vi "Trav_3D_volume.vi"(3 "Simulate/Run":T1, 5 "Traverse line":T2 {"Row Duration (mins)" format="%#.1f"; "Row No" min=0; "Trace Gas Concentration (%)" min=0.0 format="%#.2f"; "Emission Rate (l/min)" format="%#.2f"; "Tunnel Speed" format="%#.2f"; "Start X" format="%#.2f"; "Start Y" format="%#.2f"; "Start Z" format="%#.2f"; "End X" format="%#.2f"; "End Y" format="%#.2f"; "End Z" format="%#.2f"; "Averaging time (min)" min=0.0 format="%#.2f"}) -> (0 "Error Messages":string, 1 "Status":T5, 2 "Traverse line Out":T2 {"Row Duration (mins)" format="%#.1f"; "Row No" min=0; "Trace Gas Concentration (%)" min=0.0 format="%#.2f"; "Emission Rate (l/min)" format="%#.2f"; "Tunnel Speed" format="%#.2f"; "Start X" format="%#.2f"; "Start Y" format="%#.2f"; "Start Z" format="%#.2f"; "End X" format="%#.2f"; "End Y" format="%#.2f"; "End Z" format="%#.2f"; "Averaging time (min)" min=0.0 format="%#.2f"})   [LabVIEW 2011]
uses:
  Gen Trav/Multi_Run_Status.ctl
  Gen Trav/Traverse_cluster.ctl
  Gen Trav/Spacing.ctl
  Controls/Multi_run_mode.ctl
  Controls/User_Specific_mode.ctl
  Controls/Save_Data.ctl
  Controls/Setup.ctl
  ADAM Client/Sub VIs/ADAM Controls/Traverse_Level_State.ctl
  Controls/Overhead.ctl
  Globals/Trav_pos_global.vi
  Globals/Meas_global.vi
panel:
  out "Pause message":string
  in  "Pause":bool
  out "Current position":dbl[](array[numeric]) format="%.2f"
  in  "stop":bool
  in  "Array of Positions":dbl[][](array[numeric]) format="%.2f"
  out "Abcissa copy":string="Y (mm)"
  out "Abcissa":string="Y (mm)"
  in  "Plot 1":i32[](listbox)=[1]
  out "Started Profile at:":string="16/9/98 12:33"
  out "Currently on point":i32=9
  out "U":cluster{dbl[], dbl[]}[](graph)
  out "% u'/U":cluster{dbl[], dbl[]}[](graph)
  # "X           Y            Z"
  # "Start"
  # "End"
  # "X           Y            Z"
  # "Start"
  # "End"
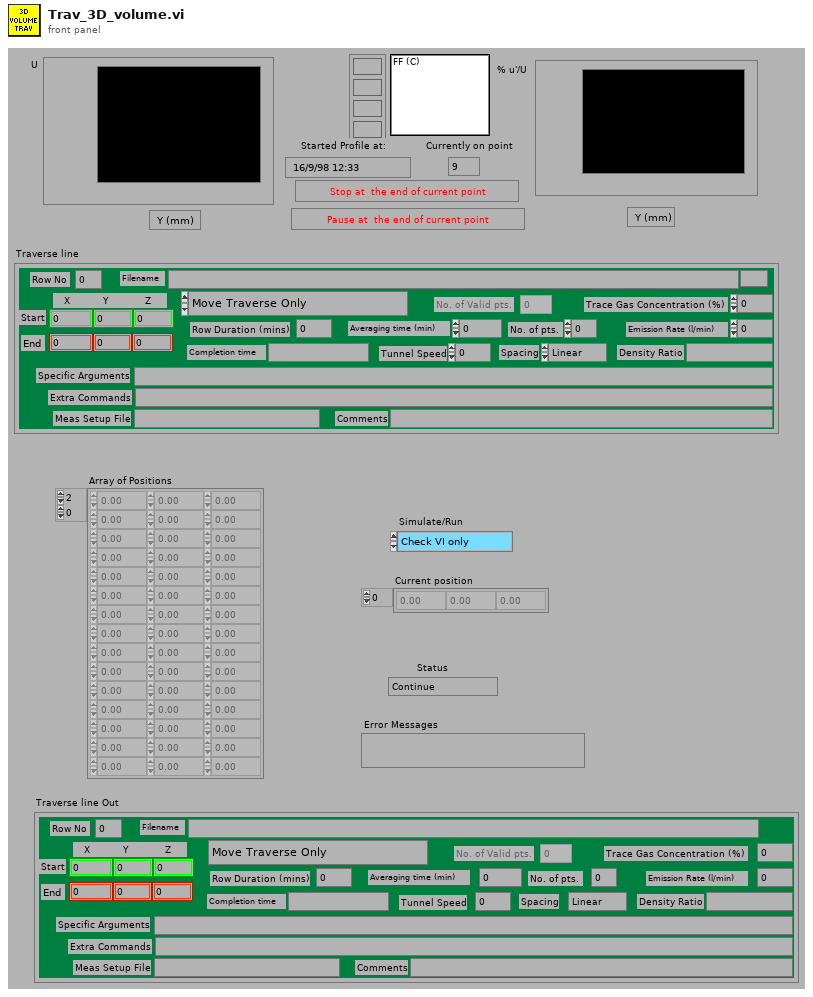
[diagram p1: front panel]
types:
  T1 = typedef "User_Specific_mode.ctl" = enum16{"Check VI only", "Run VI"}
  T2 = typedef "Traverse_cluster.ctl" = cluster{"Start X":dbl, "Start Y":dbl, "Start Z":dbl, "End X":dbl, "End Y":dbl, "End Z":dbl, "No. of pts.":i32, "Spacing":T3, "Filename":path, "Tunnel Speed":dbl, "Averaging time (min)":dbl, "Extra Commands":string, "Specific Arguments":string, "Emission Rate (l/min)":dbl, "Trace Gas Concentration (%)":dbl, "Density Ratio":string, "Comments":string, "Row No":i32, "Row Type Selector":T4, "Completion time":string, "Row Duration (mins)":dbl, "No. of Valid pts.":i32, "Meas Setup File":string}
  T3 = typedef "Spacing.ctl" = enum16{"Linear", "Log", "Gauss", "Specified", "N/A"}
  T4 = typedef "Multi_run_mode.ctl" = enum16{"Move Traverse Only", "Set Tunnel Speed Only", "Set Source Only", "Set Measurement Conditions", "Single Measurement", "Vertical Profile", "Lateral Profile", "Longitudinal Profile", "Explore Volume", "Multi-Axis Profile", "Auto Calibrate", "Meas Fast FID Bkgnd", "Check Beam Power", "Scanning Valve Measurement", "Run VI Named:", "Set ADAM Ch", "Wait (minutes)", "Send Message", "Synchronize With:", "Fall Back to this Row", "Turn Off Row Repeating", "Blank Row", "Traverse 3D Volume"}
  T5 = typedef "Multi_Run_Status.ctl" = enum16{"Continue", "Jump to Next Point", "Jump to Next Row", "Jump To Fall Back", "Terminate Run"}
  T6 = typedef "Save_Data.ctl" = enum16{"Save No Data", "Save Data"}
  T7 = typedef "Setup.ctl" = enum16{"Run Program", "Show Setup", "Save Current Setup", "Setup Front Panel"}
  T8 = typedef "Traverse_Level_State.ctl" = enum16{"Running", "Complete"}
  T9 = typedef "Overhead.ctl" = enum16{"Update total times", "Read Current Overhead", "Re Scale totals to 3 hrs", "Initialise totals to 3hr"}
  T10 = typedef "Status_Cluster.ctl" = cluster{"Status":T5, "Error Type":string, "Error Description":string}
  T11 = typedef "Velocity_cluster.ctl" = cluster{"Name":string, "U":dbl, "u^2":dbl, "u^3/(u^2)^(1.5)":dbl, "u^4/(u^2)^2 -3":dbl, "% u'/U":dbl, "Mean % Err":dbl, "u^4":dbl}
  T12 = typedef "Analysis_type_cluster.ctl" = cluster{"Analysis type":T13, "Indicies":i32[], "Name":string, "Inst Array":T14, "Info index":i32}
  T13 = typedef "Analysis_type_Enum.ctl" = enum16{"Slow Response", "Fast Response", "Weighted Fast Response", "Fast FID", "Weighted Fast FID", "Cross Wire", "Weighted Cross Wire", "Weighted LDA"}
  T14 = typedef "Instrument_Array.ctl" = enum16{"PWA", "LDA", "Analogue"}
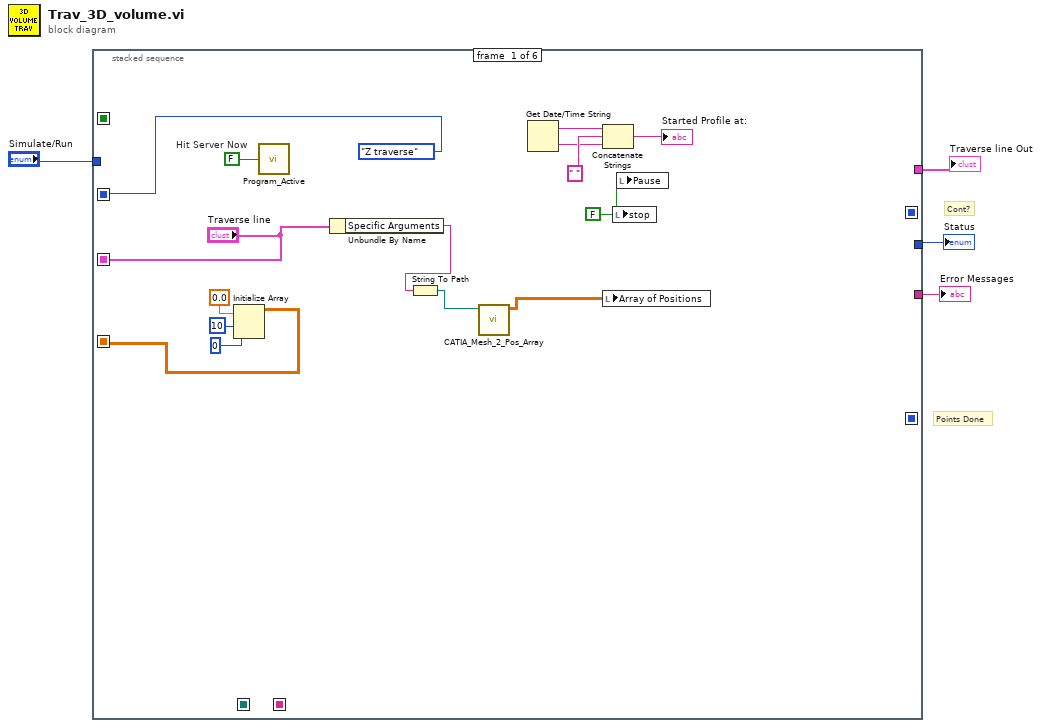
[diagram p0: block diagram]
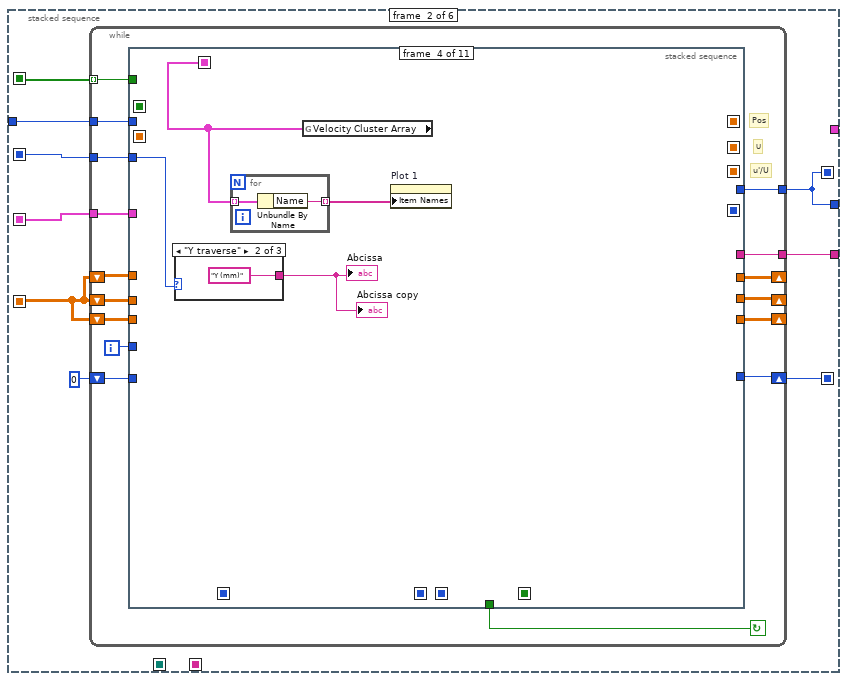
[diagram p2: hidden frame]
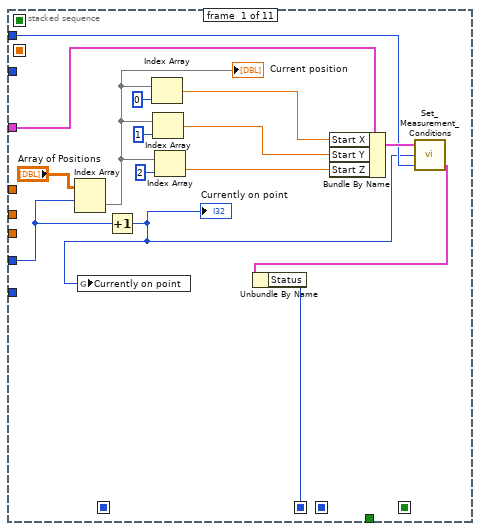
[diagram p3: hidden frame]
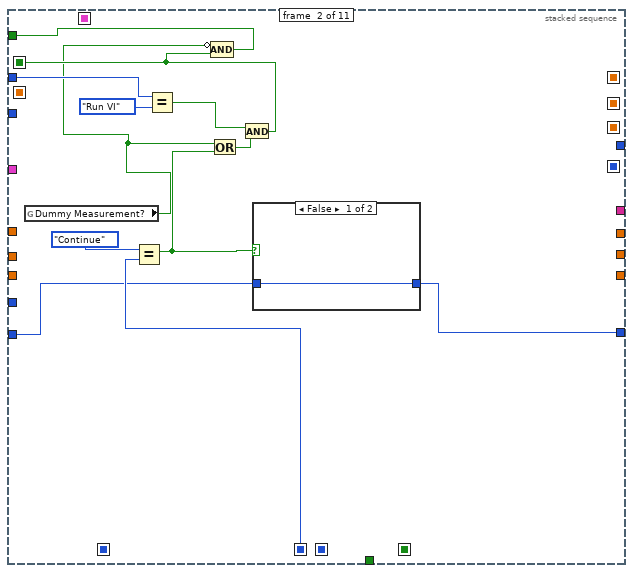
[diagram p4: hidden frame]
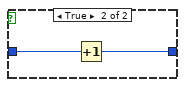
[diagram p5: hidden frame]
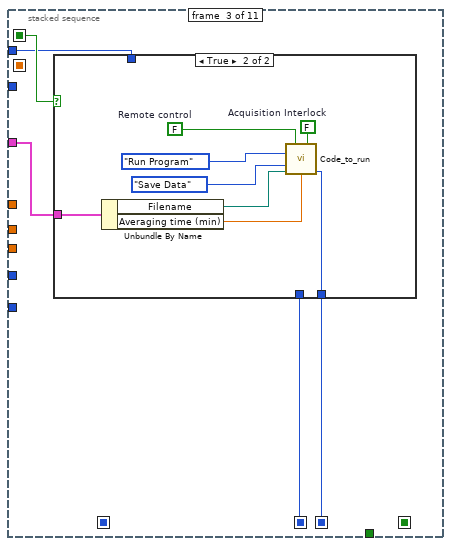
[diagram p6: hidden frame]
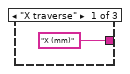
[diagram p8: hidden frame]
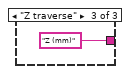
[diagram p9: hidden frame]
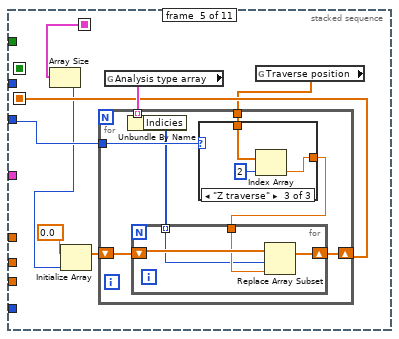
[diagram p10: hidden frame]
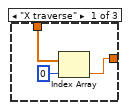
[diagram p11: hidden frame]
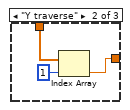
[diagram p12: hidden frame]
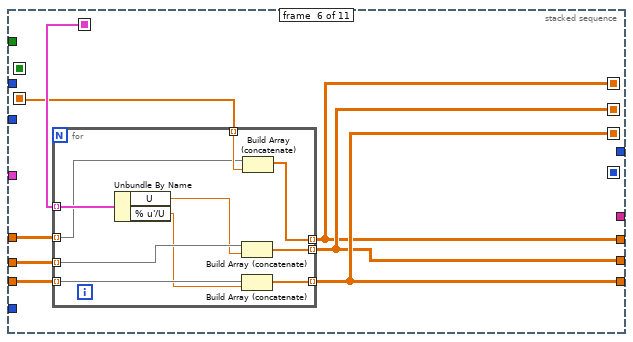
[diagram p13: hidden frame]
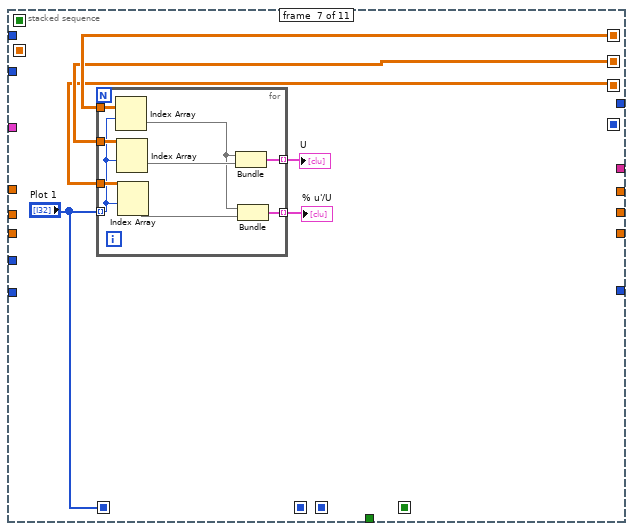
[diagram p14: hidden frame]
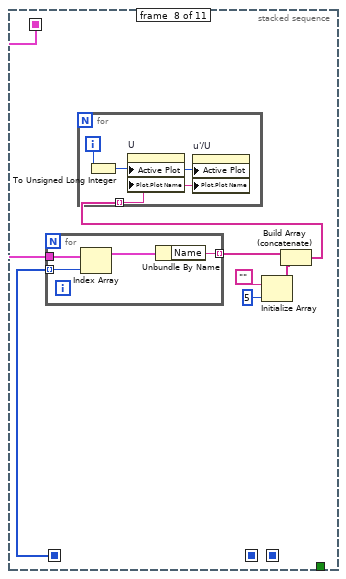
[diagram p15: hidden frame]
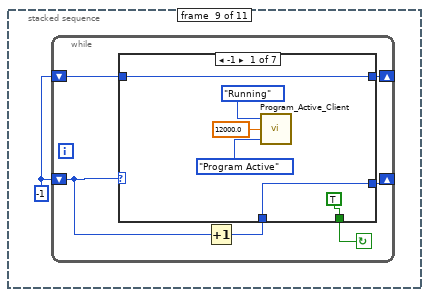
[diagram p16: hidden frame]
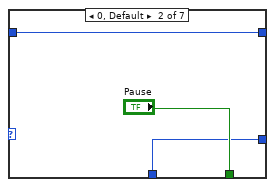
[diagram p17: hidden frame]
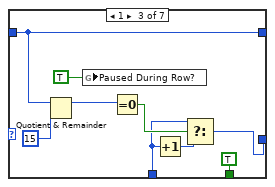
[diagram p18: hidden frame]
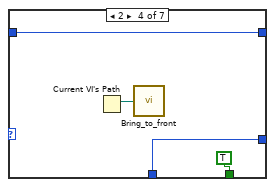
[diagram p19: hidden frame]
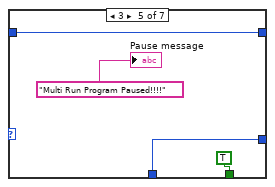
[diagram p20: hidden frame]
diagram:
  # "Points Done"
  # "Cont?"
  n1 = stacked-sequence {
    seq-local: [w12 _ _ _ _ _] -> [_ w27 _ _ _ _]
    seq-local: [enum16{"X traverse", "Y traverse", "Z traverse"}."Z traverse" ("Axis Traversed") _ _ _ _ _] -> [_ w28 _ _ _ _]
    seq-local: [_ _ w277 _ _ _] -> [_ _ _ _ w301 _]
    seq-local: [_ _ _ w284 _ _] -> [_ _ _ _ w300 _]
    seq-local: [_ w26 _ _ _ _] -> [_ _ _ _ _ _]
    seq-local: [_ w24 _ _ _ _] -> [_ _ _ w281 w299 _]
    seq-local: [_ w22 _ _ _ _] -> [_ _ _ _ _ w306]
    seq-local: ["Traverse line" _ _ _ _ _] -> [_ w21 _ _ _ w308]
    tunnel: [_ w26 _ _ _ _] -> w2
    tunnel: [_ _ _ _ _ w318] -> w4
    tunnel: "Simulate/Run" -> [_ w25 _ _ _ w317]
    tunnel: [_ w20 _ _ _ _] -> w1
    frame #0 {
      w10 = FALSE ("stop")
      w11 = FALSE  # Hit Server Now
      n2 = Initialize Array(0.0, 10, 0) -> (w12:dbl[][])
      n3 = call "Program_Active.vi"("Hit Server Now"=w11) -> ()
      n4 = Unbundle By Name("Traverse line") -> ("Specific Arguments"=w6:string)
      n5 = String To Path(string=w6) -> (path=w5:path)
      n6 = call "CATIA_Mesh_2_Pos_Array.vi"("Catia Mesh File"=w5) -> ("Array of Positions"=w8:dbl[][])  [unwired: 10 in]
      n7 = Get Date/Time String() -> (date string=w18:string, time string=w17:string)  [unwired: 3 out]
      n8 = Concatenate Strings(w18, " ", w17) -> (→"Started Profile at:":string)
      n9 = local write "Array of Positions"(w8) -> ()
      n10 = local write "stop"(w10) -> ()
      n11 = local write "Pause"(w10) -> ()
    }
    frame #1 {
      n12 = while {
        shift-left: 0 -> [w31]
        shift-right: [w30] -> w22
        tunnel: [w32] -> w24 mode=indexing
        tunnel: w21 -> [w33]
        tunnel: w25 -> [w34]
        tunnel: [w35] -> w26
        shift-left: w27 -> [w38]
        shift-right: [w37] -> _
        tunnel: w28 -> [w39]
        shift-left: w27 -> [w41]
        shift-right: [w40] -> _
        shift-left: w27 -> [w43]
        shift-right: [w42] -> _
        tunnel: [w29] -> w20
        i -> [w44]
        stop <- w36 continue-if-true
        # "Pos"
        # "U"
        # "u'/U"
        n13 = stacked-sequence {
          seq-local: [_ _ _ _ w103 _ _ _ _ _ _] -> [_ _ _ _ _ w128 _ _ _ _ _]
          seq-local: [_ _ _ w92 _ _ _ _ _ _ _] -> [_ _ _ _ w102 w131 _ w159 _ _ _]
          seq-local: [_ _ _ _ _ w126 _ _ _ _ _] -> [_ _ _ _ _ _ w149 _ _ _ _]
          seq-local: [_ _ _ _ _ w129 _ _ _ _ _] -> [_ _ _ _ _ _ w148 _ _ _ _]
          seq-local: [_ _ _ _ _ w130 _ _ _ _ _] -> [_ _ _ _ _ _ w147 _ _ _ _]
          seq-local: [_ _ _ _ _ _ "Plot 1" _ _ _ _] -> [_ _ _ _ _ _ _ w165 _ _ _]
          seq-local: [_ _ w78 _ _ _ _ _ _ _ _] -> [_ _ _ _ _ _ _ _ _ w223 _]
          seq-local: [w49 _ _ _ _ _ _ _ _ _ _] -> [_ w69 w76 _ _ _ _ _ _ _ _]
          seq-local: [_ w62 _ _ _ _ _ _ _ _ _] -> [_ _ w77 _ _ _ _ _ _ _ _]
          seq-local: [_ _ _ _ _ _ _ _ _ w218 _] -> [_ _ _ _ _ _ _ _ _ _ w239]
          seq-local: [_ _ _ _ _ _ _ _ _ w217 _] -> [_ _ _ _ _ _ _ _ _ _ w233]
          tunnel: w44 -> [w46 _ _ _ _ _ _ _ _ w229 w236]
          tunnel: w43 -> [_ _ _ _ _ w133 _ _ _ _ _]
          tunnel: [_ _ _ _ _ w129 _ _ _ _ _] -> w42
          tunnel: w41 -> [_ _ _ _ _ w132 _ _ _ _ _]
          tunnel: [_ _ _ _ _ w130 _ _ _ _ _] -> w40
          tunnel: w39 -> [_ _ _ w90 w104 _ _ _ _ _ _]
          tunnel: w38 -> [_ _ _ _ _ w127 _ _ _ _ _]
          tunnel: [_ _ _ _ _ w126 _ _ _ _ _] -> w37
          tunnel: [_ _ _ _ _ _ _ _ _ w218 _] -> w36
          tunnel: w33 -> [w53 _ w79 _ _ _ _ _ _ _ w237]
          tunnel: [_ _ _ _ _ _ _ _ _ _ w235] -> w35
          tunnel: w34 -> [w51 w71 w75 _ _ _ _ _ _ _ w238]
          tunnel: [_ w61 _ _ _ _ _ _ _ _ _] -> w32
          tunnel: w31 -> [_ w66 _ _ _ _ _ _ _ _ _]
          tunnel: [_ w65 _ _ _ _ _ _ _ _ _] -> w30
          tunnel: [_ _ _ _ _ _ _ _ _ _ w234] -> w29
          frame #0 {
            n14 = Index Array(array="Array of Positions", index (row)=w46) -> (element=w45:dbl[])  [unwired: 1 in]
            "Current position" <- w45
            n15 = Increment(x=w46) -> (x+1=w48:i32)
            "Currently on point" <- w48
            n16 = global write "Trav_pos_global.vi" "Currently on point"(w48) -> ()
            n17 = Index Array(array=w45, index=0 ("Index")) -> (element=w56:dbl)
            n18 = Index Array(array=w45, index=1 ("Index")) -> (element=w55:dbl)
            n19 = Index Array(array=w45, index=2 ("Index")) -> (element=w54:dbl)
            n20 = Bundle By Name(cluster=w53, "Start X"=w56, "Start Y"=w55, "Start Z"=w54) -> (w52:T2)
            n21 = call "Set_Measurement_Conditions.vi"("Simulate/Run"=w51, "Currently on Point"=w48, "Traverse line"=w52) -> ("Status Cluster"=w50:T10)  [unwired: 2 out]
            n22 = Unbundle By Name(w50) -> ("Status"=w49:T5)
          }
          frame #1 {
            n23 = global read "Trav_pos_global.vi" "Dummy Measurement?"() -> (w60:bool)
            n24 = Equal?(x=Multi_Run_Status."Continue" ("Status"), y=w69) -> (x = y?=w64:bool)
            n25 = Equal?(x=w71, y=User_Specific_mode."Run VI" ("Simulate/Run")) -> (x = y?=w67:bool)
            n26 = Or(x=w60, y=w64) -> (x .or. y?=w63:bool)
            n27 = And(x=w67, y=w63) -> (x .and. y?=w62:bool)
            n28 = Compound Arithmetic op=AND(invert w60, w62) -> (w61:bool)
            n29 = case shown="False" w64 {
              tunnel: w66 -> [w72 w74]
              tunnel: [w72 w73] -> w65
              frame False {
              }
              frame True {
                n30 = Increment(x=w74) -> (x+1=w73:i32)
              }
            }
          }
          frame #2 {
            n31 = case shown="True" w77 {
              tunnel: w79 -> [_ w88]
              tunnel: [w80 w87] -> w78
              tunnel: w76 -> [w80 _]
              tunnel: w75 -> [_ _]
              frame False {
              }
              frame True {
                w83 = FALSE  # Acquisition Interlock
                w86 = FALSE  # Remote control
                n32 = Unbundle By Name(w88) -> ("Filename"=w84:path, "Averaging time (min)"=w85:dbl)
                n33 = call "Code_to_run.vi"("Acquisition Interlock"=w83, "setup"=Setup."Run Program", "Remote control"=w86, "File"=Save_Data."Save Data", "Results Filename"=w84, "Averaging time (min)"=w85) -> ("Status"=w87:T5)  [unwired: 5 in, 4 out]
              }
            }
          }
          frame #3 {
            n34 = case shown="\"Y traverse\"" w90 {
              tunnel: ["X (mm)" "Y (mm)" "Z (mm)"] -> w89
              frame "X traverse" {
              }
              frame "Y traverse" {
              }
              frame "Z traverse" {
              }
            }
            "Abcissa" <- w89
            "Abcissa copy" <- w89
            n35 = global read "Meas_global.vi" "Velocity Cluster Array"() -> (w92:T11[])
            n36 = for {
              tunnel: w92 -> [w97] mode=indexing
              tunnel: [w96] -> w91 mode=indexing
              n37 = Unbundle By Name(w97) -> ("Name"=w96:string)
            }
            n38 = property on="Plot 1" class="LstBox (strict)"("Item Names"=w91) -> ()  [unwired: 2 in, 2 out]
          }
          frame #4 {
            n39 = Array Size(array=w102) -> (size(s)=w101:i32)
            n40 = Initialize Array(0.0, w101) -> (w99:dbl[])
            n41 = global read "Meas_global.vi" "Analysis type array"() -> (w105:T12[])
            n42 = global read "Trav_pos_global.vi" "Traverse position"() -> (w98:dbl[])
            n43 = for {
              shift-right: [w109] -> w103
              shift-left: w99 -> [w110]
              tunnel: w105 -> [w112] mode=indexing
              tunnel: w104 -> [w111]
              tunnel: w98 -> [w106]
              n44 = Unbundle By Name(w112) -> ("Indicies"=w107:i32[])
              n45 = case shown="\"Z traverse\"" w111 {
                tunnel: [w118 w121 w123] -> w108
                tunnel: w106 -> [w119 w120 w124]
                frame "X traverse" {
                  n46 = Index Array(array=w119, index=0) -> (element=w118:dbl)
                }
                frame "Y traverse" {
                  n47 = Index Array(array=w120, index=1) -> (element=w121:dbl)
                }
                frame "Z traverse" {
                  n48 = Index Array(array=w124, index=2) -> (element=w123:dbl)
                }
              }
              n49 = for {
                shift-right: [w115] -> w109
                shift-left: w110 -> [w116]
                tunnel: w108 -> [w114]
                tunnel: w107 -> [w113] mode=indexing
                n50 = Replace Array Subset(array=w116, new element=w114, index=w113) -> (w115:dbl[])
              }
            }
          }
          frame #5 {
            n51 = for {
              tunnel: w133 -> [w143] mode=indexing
              tunnel: [w141] -> w129 mode=indexing
              tunnel: w132 -> [w140] mode=indexing
              tunnel: [w138] -> w130 mode=indexing
              tunnel: w131 -> [w137] mode=indexing
              tunnel: w128 -> [w136] mode=indexing
              tunnel: w127 -> [w135] mode=indexing
              tunnel: [w134] -> w126 mode=indexing
              n52 = Unbundle By Name(w137) -> ("U"=w142:dbl, "% u'/U"=w139:dbl)
              n53 = Build Array (concatenate)(w143, w142) -> (w141:dbl[])
              n54 = Build Array (concatenate)(w140, w139) -> (w138:dbl[])
              n55 = Build Array (concatenate)(w135, w136) -> (w134:dbl[])
            }
          }
          frame #6 {
            n56 = for {
              tunnel: "Plot 1" -> [w150] mode=indexing
              tunnel: w149 -> [w158]
              tunnel: w148 -> [w157]
              tunnel: w147 -> [w156]
              tunnel: [w152] -> w146 mode=indexing
              tunnel: [w151] -> w145 mode=indexing
              n57 = Index Array(array=w158, index (row)=w150) -> (element=w154:dbl[])  [unwired: 1 in]
              n58 = Index Array(array=w157, index (row)=w150) -> (element=w155:dbl[])  [unwired: 1 in]
              n59 = Index Array(array=w156, index (row)=w150) -> (element=w153:dbl[])  [unwired: 1 in]
              n60 = Bundle(w154, w155) -> (w151:cluster{dbl[], dbl[]})  [unwired: 1 out]
              n61 = Bundle(w154, w153) -> (w152:cluster{dbl[], dbl[]})  [unwired: 1 out]
            }
            "U" <- w145
            "% u'/U" <- w146
          }
          frame #7 {
            n62 = for {
              tunnel: w165 -> [w169] mode=indexing
              tunnel: w159 -> [w167]
              tunnel: [w166] -> w162 mode=indexing
              n63 = Index Array(array=w167, index=w169) -> (element=w168:T11)
              n64 = Unbundle By Name(w168) -> ("Name"=w166:string)
            }
            n65 = Initialize Array("", 5) -> (w161:string[])
            n66 = Build Array (concatenate)(w162, w161) -> (w160:string[])
            n67 = for {
              tunnel: w160 -> [w170] mode=indexing
              i -> [w172]
              n68 = To Unsigned Long Integer(number=w172) -> (unsigned 32bit integer=w171:u32)
              n69 = property on="U" class="XYGraph (strict)"("Active Plot"=w171, "Plot.Plot Name"=w170) -> ()  [unwired: 2 in, 2 out]
              n70 = property on="u'/U" class="XYGraph (strict)"("Active Plot"=w171, "Plot.Plot Name"=w170) -> ()  [unwired: 2 in, 2 out]
            }
          }
          frame #8 {
            w173 = -1
            n71 = while {
              shift-left: w173 -> [w174]
              shift-right: [w175] -> _
              shift-left: w173 -> [w178]
              shift-right: [w179] -> _
              stop <- w176 continue-if-true
              n72 = Increment(x=w178) -> (x+1=w177:i32)
              n73 = case shown="-1" w178 {
                tunnel: [w184 w187 w191 w201 w204 w208 0] -> w179
                tunnel: w177 -> [w184 w187 w193 w201 w204 w208 _]
                tunnel: [TRUE ("Pause") "Pause" TRUE ("Pause") TRUE ("Pause") TRUE ("Pause") TRUE ("Pause") TRUE ("Pause")] -> w176
                tunnel: [w183 w186 w189 w198 w202 w206 w211] -> w175
                tunnel: w174 -> [w183 w186 w189 w198 w202 w206 w212]
                frame -1 {
                  n74 = call "Program_Active_Client.vi"("Mode"=enum16{"Program Active", "Traverse Level State"}."Program Active", "Time till next contact (Sec)"=12000.0, "Traverse level State"=Traverse_Level_State."Running") -> ()  [unwired: 3 out]
                }
                frame 0, Default {
                }
                frame 1 {
                  n75 = Quotient & Remainder(x=w189, y=15) -> (x-y*floor(x/y)=w195:i32)  [unwired: 1 out]
                  n76 = global write "Trav_pos_global.vi" "Paused During Row?"(TRUE ("Paused During Row?")) -> ()
                  n77 = Equal To 0?(x=w195) -> (x = 0?=w194:bool)
                  n78 = Increment(x=w193) -> (x+1=w192:i32)
                  n79 = Select(t=w193, s=w194, f=w192) -> (s? t:f=w191:i32)
                }
                frame 2 {
                  n80 = Current VI's Path() -> (path=w199:path)
                  n81 = call "Bring_to_front.vi"("path"=w199) -> ()
                }
                frame 3 {
                  "Pause message" <- "Multi Run Program Paused!!!!" ("Pause message")
                }
                frame 4 {
                  n82 = property on="Pause message" class="Str"("Visible"=TRUE) -> ()  [unwired: 2 in, 2 out]
                  n83 = Wait Until Next ms Multiple(millisecond multiple=u32 1500) -> ()  [unwired: 1 out]
                }
                frame 5 {
                  n84 = Increment(x=w212) -> (x+1=w211:i32)
                  n85 = property on="Pause message" class="Str"("Visible"=FALSE) -> ()  [unwired: 2 in, 2 out]
                  n86 = Wait Until Next ms Multiple(millisecond multiple=u32 1500) -> ()  [unwired: 1 out]
                }
              }
            }
          }
          frame #9 {
            n87 = Increment(x=w229) -> (x+1=w228:i32)
            n88 = local read "Array of Positions"() -> (w219:dbl[][])
            n89 = case shown="\"Jump to Next Point\"" w223 {
              tunnel: [TRUE TRUE FALSE] -> w226
              frame "Continue" {
              }
              frame "Jump to Next Point" {
              }
              frame "Jump to Next Row", Default {
              }
            }
            n90 = Array Size(array=w219) -> (size(s)=w222:i32[])
            n91 = Index Array(array=w222, index=0 ("Index")) -> (element=w220:i32)
            n92 = Less?(x=w228, y=w220) -> (x < y?=w227:bool)
            n93 = Compound Arithmetic op=AND(w226, invert "stop", w227) -> (w218:bool)
            n94 = Select(t=Multi_Run_Status."Terminate Run" ("Status"), s="stop", f=w223) -> (s? t:f=w217:T5)
          }
          frame #10 {
            n95 = case shown="True" w239 {
              tunnel: w238 -> [_ w248]
              tunnel: w237 -> [_ w247]
              tunnel: w236 -> [_ w246]
              tunnel: [w241 w243] -> w235
              tunnel: ["" w242] -> w234
              tunnel: w233 -> [w241 _]
              frame False {
              }
              frame True {
                n96 = case shown="\"Check VI only\"" w248 {
                  tunnel: w247 -> [w264 _]
                  tunnel: w246 -> [w259 _]
                  tunnel: [w249 timestamp(0 s since 1904-01-01)] -> w245
                  frame "Check VI only" {
                    n97 = Increment(x=w259) -> (x+1=w257:i32)
                    n98 = Unbundle By Name(w264) -> ("Averaging time (min)"=w261:dbl)
                    n99 = global read "Trav_pos_global.vi" "Simulation Time"() -> (w251:timestamp)
                    n100 = To Double Precision Float(number=w251) -> (double precision float=w252:dbl)
                    n101 = Multiply(x=60.0, y=w261) -> (x*y=w260:dbl)
                    n102 = Add(x=w260, y=10.0 ("Scalable Time (Sec)")) -> (x+y=w258:dbl)
                    n103 = Multiply(x=w258, y=w257) -> (x*y=w255:dbl)
                    n104 = call "Overhead_Factor.vi"("Mode"=Overhead."Read Current Overhead") -> ("Current Overhead Factor"=w256:dbl)  [unwired: 3 in]
                    n105 = Multiply(x=w256, y=w255) -> (x*y=w253:dbl)
                    n106 = Add(x=w252, y=w253) -> (x+y=w250:dbl)
                    n107 = To Time Stamp(1:w250) -> (0:w249:timestamp)
                  }
                  frame "Run VI" {
                  }
                }
                n108 = call "Run_FFID_Bkgnd.vi"("Simulated Time"=w245, "Run Now?"=FALSE, "Simulate/Run"=w248) -> ("Error Messages"=w242:string, "Status"=w243:T5)  [unwired: 1 out]
              }
            }
          }
        }
      }
    }
    frame #2 {
      n109 = global read "Meas_global.vi" "Start Time of experiment"() -> (w267:dbl)
      n110 = global read "Meas_global.vi" "Raw data file"() -> (w279:path)
      n111 = Strip Path(path=w279) -> (stripped path=w278:path)  [unwired: 1 out]
      n112 = call "Sec_to_date_filename.vi"("seconds"=w267) -> ("Day"=w269:string, "Time"=w270:string)  [unwired: 2 out]
      n113 = Format Into String(format string="Cmd_%s_%s.xls", w269, w270) -> (resulting string=w272:string)  [unwired: 2 in, 1 out]
      n114 = call "Fast_string_Replace.vi"("Replace match with:"="-", "Input String"=w272, "regular expression"=":") -> ("Output String"=w275:string)  [unwired: 2 out]
      n115 = call "Fast_string_Replace.vi"("Replace match with:"="", "Input String"=w275, "regular expression"=" ") -> ("Output String"=w266:string)  [unwired: 2 out]
      n116 = Build Path(base path=w278, name or relative path=w266) -> (appended path=w277:path)
    }
    frame #3 {
      w290 = "\t"
      n117 = local read "Array of Positions"() -> (w283:dbl[][])
      n118 = Number To Fractional String(number=w283, precision (6)=i16 2) -> (F-format string=w282:string[][])  [unwired: 2 out]
      n119 = for {
        tunnel: w282 -> [w295] mode=indexing
        tunnel: w281 -> [w294] mode=indexing
        tunnel: [w292] -> w280 mode=indexing
        n120 = case shown="False" w294 {
          tunnel: ["Unobtainable Position" ""] -> w293
          frame False {
          }
          frame True {
          }
        }
        n121 = Build Array (concatenate)(w295, w293) -> (w292:string[])
      }
      n122 = Concatenate Strings("X", w290, "Y", w290, "Z") -> (w285:string)
      n123 = call "2D_array_to_string.vi"("2D data array"=w280, "Column titles  (separated by tabs)"=w285, "Array title"="Requested positions") -> ("Output string"=w284:string)
    }
    frame #4 {
      n124 = Or Array Elements(Boolean array=w299) -> (logical OR=w298:bool)
      n125 = case shown="True" w298 {
        tunnel: w301 -> [_ w304]
        tunnel: w300 -> [_ w302]
        frame False {
        }
        frame True {
          w303 = FALSE  # Lock File
          w305 = TRUE  # append to file? (new file:F)
          n126 = call "Write_Characters_To_File.vi"("file path (dialog if empty)"=w304, "character string"=w302, "append to file? (new file:F)"=w305, "Lock File"=w303) -> ()  [unwired: 1 in, 4 out]
        }
      }
    }
    frame #5 {
      n127 = local read "Array of Positions"() -> (w310:dbl[][])
      n128 = Array Size(array=w310) -> (size(s)=w312:i32[])
      n129 = Index Array(array=w312, index=0 ("Index")) -> (element=w309:i32)
      n130 = Bundle By Name(cluster=w308, "No. of Valid pts."=w306) -> (w307:T2)
      n131 = Not Equal?(x=w309, y=w306) -> (x != y?=w315:bool)
      n132 = Equal?(x=User_Specific_mode."Run VI" ("Simulate/Run"), y=w317) -> (x = y?=w314:bool)
      n133 = And(x=w314, y=w315) -> (x .and. y?=w313:bool)
      n134 = case shown="True" w313 {
        tunnel: w307 -> [w319 w331]
        tunnel: [w319 w330] -> w318
        tunnel: w306 -> [_ w329]
        frame False {
        }
        frame True {
          w320 = " !!Program added comments"
          n135 = Unbundle By Name(w331) -> ("Comments"=w321:string)
          n136 = Equal To 0?(x=w329) -> (x = 0?=w328:bool)
          n137 = Match Pattern(string=w321, regular expression=w320) -> (match substring=w323:string)  [unwired: 4 out]
          n138 = Select(t=" !!(Row Skipped)", s=w328, f=" !!(Row Partially Skipped)") -> (s? t:f=w324:string)
          n139 = Empty String/Path?(string/path=w323) -> (empty?=w322:bool)
          n140 = case shown="True" w322 {
            tunnel: [w334 w338] -> w325
            tunnel: w324 -> [w333 w337]
            tunnel: w320 -> [_ w336]
            tunnel: w321 -> [w332 w335]
            frame False {
              n141 = Concatenate Strings(w332, w333) -> (w334:string)
            }
            frame True {
              n142 = Concatenate Strings(w335, w336, w337) -> (w338:string)
            }
          }
          n143 = Bundle By Name(cluster=w331, "Comments"=w325) -> (w330:T2)
        }
      }
    }
  }
  "Status" <- w2
  "Traverse line Out" <- w4
  "Error Messages" <- w1
